vi "LHe transfer readiness.vi"() -> ()   [LabVIEW 2024]
panel:
  out "Transfer time (s)":dbl=13.499
  in  "wait after transfer (s)":dbl=300.0
  in  "done":bool
  out "Message":string="Please press  Initiate LHe transfer button before starting LHe transfer."
  in  "initiate":bool=TRUE
  out "condition met":i32=5
  in  "VIs to pause":string[](array[string])=["ThermalHall.vi", "MonoVu.vi"]
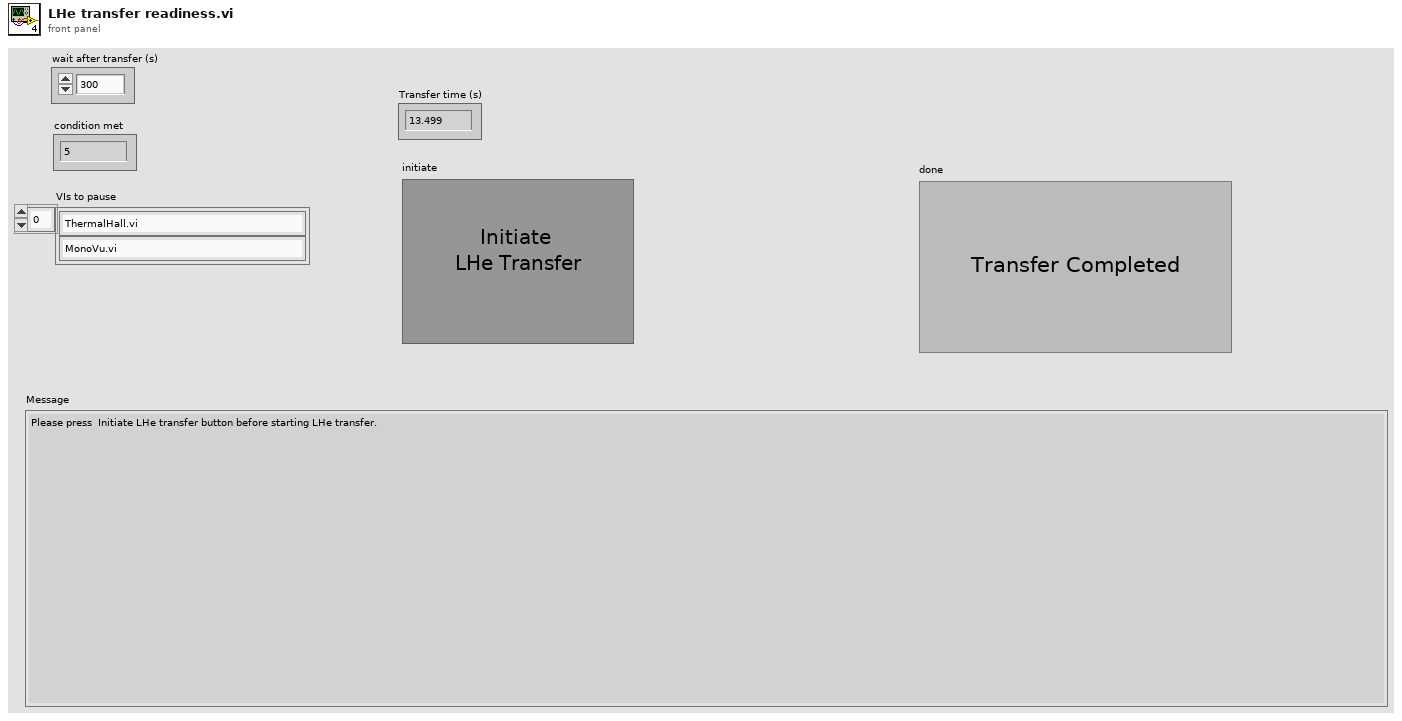
[diagram p1: front panel]
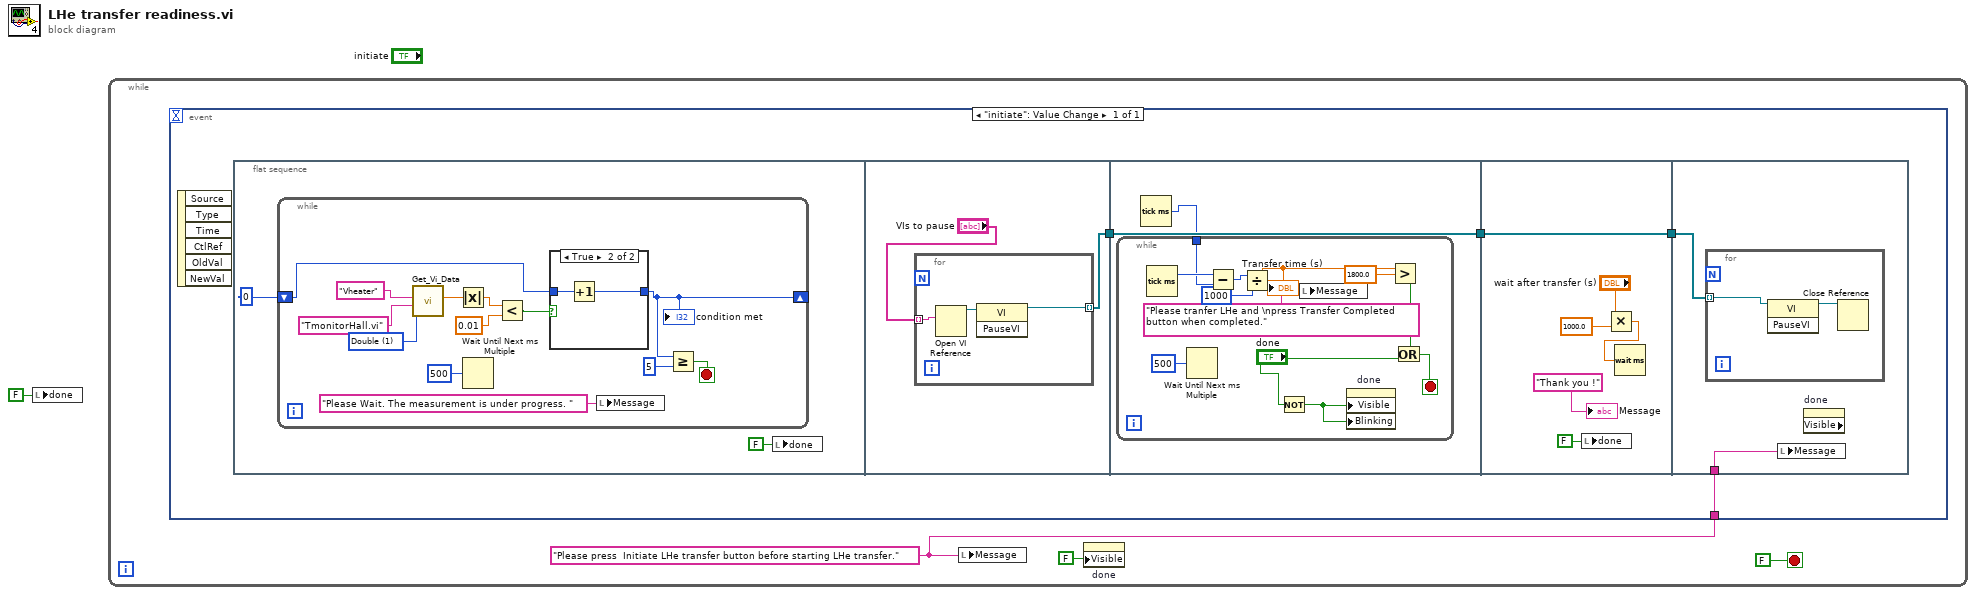
[diagram p0: block diagram]
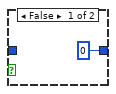
[diagram p2: hidden frame]
diagram:
  n1 = local write "done"(FALSE ("done")) -> ()
  n2 = while {
    stop <- FALSE stop-if-true
    w2 = "Please press  Initiate LHe transfer button before starting LHe transfer." ("Message")
    n3 = event shown="[0] \"initiate\": Value Change" {
      selector: _ -> [_]
      dyn-events: _ -> [_]
      timeout: _ -> [_]
      tunnel: w2 -> [w5]
      event "initiate": Value Change {
        n4 = event-data() -> ()  [unwired: 1 in, 6 out]
        n5 = flat-sequence {
          tunnel: [w27] -> w6
          tunnel: [w33] -> w7
          tunnel: w6 -> [w33]
          tunnel: [w48] -> w8
          tunnel: w7 -> [w48]
          tunnel: w8 -> [w53]
          tunnel: w5 -> [w52]
          frame #0 {
            n6 = while {
              shift-right: [w15] -> _
              shift-left: 0 -> [w16]
              stop <- w13 stop-if-true
              w21 = u16 1 items=["String", "Double", "Boolean", "Variant"] ("Data Type")
              n7 = call "Get_Vi_Data.vi"("Data Type"=w21, "VI name"="TmonitorHall.vi", "Control Name"="Vheater") -> ("Data (Double)"=w20:dbl)  [unwired: 4 in, 4 out]
              n8 = Absolute Value(x=w20) -> (abs(x)=w19:dbl)
              n9 = Wait Until Next ms Multiple(millisecond multiple=u32 500) -> ()  [unwired: 1 out]
              n10 = Less?(x=w19, y=0.01) -> (x < y?=w17:bool)
              n11 = case shown="True" w17 {
                tunnel: [0 w25] -> w15
                tunnel: w16 -> [_ w26]
                frame False {
                }
                frame True {
                  n12 = Increment(x=w26) -> (x+1=w25:i32)
                }
              }
              "condition met" <- w15
              n13 = local write "Message"("Please Wait. The measurement is under progress. " ("String")) -> ()
              n14 = Greater Or Equal?(x=w15, y=5) -> (x >= y?=w13:bool)
            }
            n15 = local write "done"(FALSE ("done")) -> ()
          }
          frame #1 {
            n16 = for {
              tunnel: "VIs to pause" -> [w31] mode=indexing
              tunnel: [w29] -> w27 mode=indexing
              n17 = Open VI Reference(vi path=w31) -> (vi reference=w30:refnum<vi>)  [unwired: 5 in, 1 out]
              n18 = invoke class="VI" method="PauseVI"(reference=w30) -> (reference out=w29:refnum<vi>)  [unwired: 2 in, 2 out]
            }
          }
          frame #2 {
            n19 = Tick Count (ms)() -> (millisecond timer value=w32:u32)
            n20 = while {
              tunnel: w32 -> [w41]
              stop <- w34 stop-if-true
              n21 = Tick Count (ms)() -> (millisecond timer value=w42:u32)
              n22 = Wait Until Next ms Multiple(millisecond multiple=u32 500) -> ()  [unwired: 1 out]
              n23 = Subtract(x=w42, y=w41) -> (x-y=w40:u32)
              n24 = Divide(x=w40, y=u32 1000) -> (x/y=w38:dbl)
              "Transfer time (s)" <- w38
              n25 = Not(x="done") -> (.not. x?=w43:bool)
              n26 = local write "Message"("Please tranfer LHe and \npress Transfer Completed button when completed." ("String")) -> ()
              n27 = property on="done" class="Bool (strict)"("Visible"=w43, "Blinking"=w43) -> ()  [unwired: 2 in, 2 out]
              n28 = Greater?(x=w38, y=1800.0) -> (0:w35:bool)
              n29 = Or(x=w35, y="done") -> (x .or. y?=w34:bool)
            }
          }
          frame #3 {
            n30 = local write "done"(FALSE ("done")) -> ()
            n31 = Multiply(x="wait after transfer (s)", y=1000.0) -> (x*y=w49:dbl)
            n32 = Wait (ms)(milliseconds to wait=w49) -> ()  [unwired: 1 out]
            "Message" <- "Thank you !" ("String")
          }
          frame #4 {
            n33 = for {
              tunnel: w53 -> [w54] mode=indexing
              n34 = invoke class="VI" method="PauseVI"(reference=w54) -> (reference out=w55:refnum<vi>)  [unwired: 2 in, 2 out]
              n35 = Close Reference(reference=w55) -> ()  [unwired: 1 in, 1 out]
            }
            n36 = local write "Message"(w52) -> ()
            n37 = property on="done" class="Bool (strict)" props=["Visible"]() -> ()  [unwired: 2 in, 3 out]
          }
        }
      }
    }
    n38 = local write "Message"(w2) -> ()
    n39 = property on="done" class="Bool (strict)"("Visible"=FALSE) -> ()  [unwired: 2 in, 2 out]
  }
